vi "Get%20Printers%20Available%20and%20Setting%20a%20Default%20One%202012%20NIVerified.vi"() -> ()   [LabVIEW 2015]
uses:
  System.Drawing
  winspool.drv
panel:
  out "error out":errorcluster
  out "Printers":T1(array[cluster])
  in  "Index":i32
  # "Overview:This example shows a quick way to provide the user a list of print available and set a default one.\nRequirements:\n•\tLabVIEW 2012 (or compatible)\nInstructions:\n•\tSelect the printer number as the default one.\n•\tRun the program"
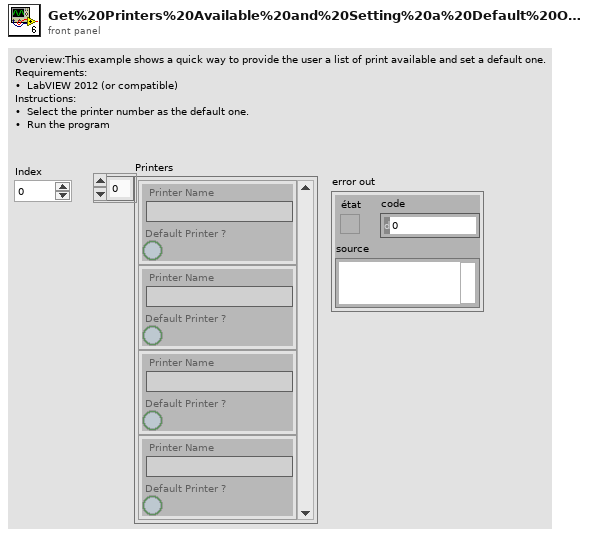
[diagram p1: front panel]
types:
  T1 = cluster{"Printer Name":string, "Default Printer ?":bool}[]
  T2 = cluster{"get_Item":string, "IsDefaultPrinter":bool}
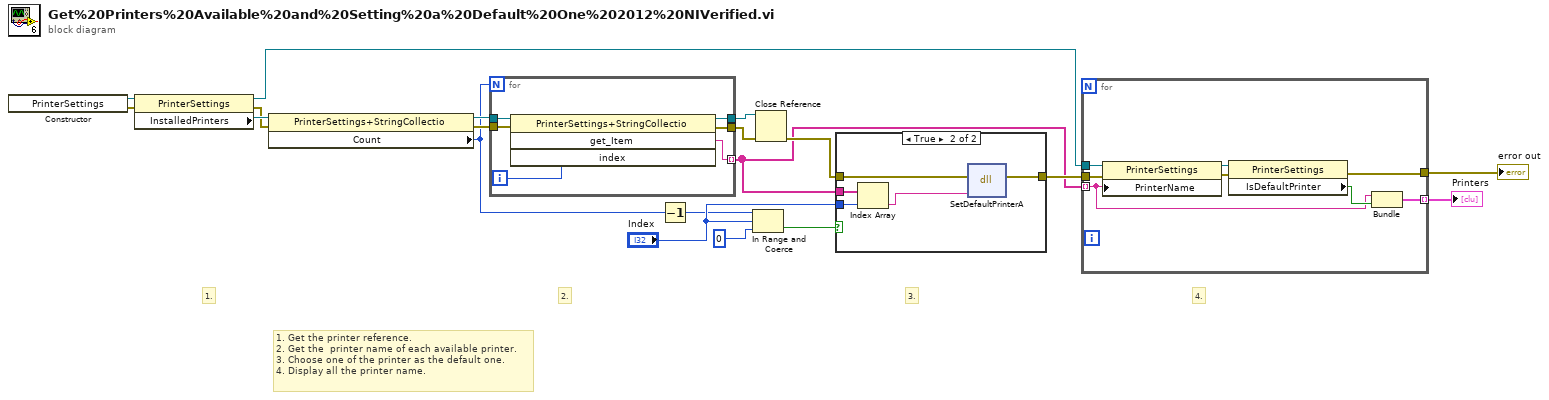
[diagram p0: block diagram]
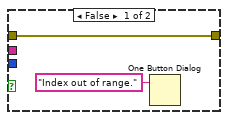
[diagram p2: hidden frame]
diagram:
  # "1. Get the printer reference.\n2. Get the  printer name of each available printer.\n3. Choose one of the printer as the default one.\n4. Display all the printer name."
  # "4."
  # "3."
  # "2."
  # "1."
  n1 = constructor class="PrinterSettings"() -> (reference out=w13:refnum<k24>, error out=w16:errorcluster)  [unwired: 3 in, 1 out]
  n2 = property class="PrinterSettings"(reference=w13, error in=w16) -> (reference out=w4:refnum<k24>, error out=w15:errorcluster, "InstalledPrinters"=w19:refnum<k24>)
  n3 = property class="PrinterSettings+StringCollectio"(reference=w19, error in=w15) -> (reference out=w17:refnum<k24>, error out=w14:errorcluster, "Count"=w7:i32)
  n4 = for {
    N: w7 -> [_]
    tunnel: w17 -> [w25]
    tunnel: [w20] -> w3 mode=indexing
    tunnel: [w23] -> w18
    tunnel: [w22] -> w12
    tunnel: w14 -> [w21]
    i -> [w24]
    n5 = invoke class="PrinterSettings+StringCollectio" method="get_Item"(reference=w25, error in=w21, "index"=w24) -> (reference out=w23:refnum<k24>, error out=w22:errorcluster, "get_Item"=w20:string)  [unwired: 1 in, 1 out]
  }
  n6 = Decrement(x=w7) -> (x-1=w8:i32)
  n7 = In Range and Coerce(upper limit=w8, x="Index", lower limit=0 ("limite inférieure")) -> (In Range?=w11:bool)  [unwired: 1 out]
  n8 = Close Reference(reference=w18, error in (no error)=w12) -> (error out=w5:errorcluster)
  n9 = case shown="True" w11 {
    tunnel: w3 -> [_ w32]
    tunnel: "Index" -> [_ w31]
    tunnel: [w26 w29] -> w6
    tunnel: w5 -> [w26 w28]
    frame False {
      n10 = One Button Dialog(message="Index out of range.") -> ()  [unwired: 1 in, 1 out]
    }
    frame True {
      n11 = Index Array(array=w32, index=w31) -> (element=w30:string)
      n12 = dll-call lib="winspool.drv" fn="SetDefaultPrinterA"(error in=w28, "pszPrinter"=w30) -> (error out=w29:errorcluster)  [unwired: 4 in, 1 out]
    }
  }
  n13 = for {
    tunnel: w6 -> [w35]
    tunnel: [w37] -> w2 mode=indexing
    tunnel: w4 -> [w36]
    tunnel: w3 -> [w34] mode=indexing
    tunnel: [w33] -> w1
    n14 = property class="PrinterSettings"(reference=w36, error in=w35, "PrinterName"=w34) -> (reference out=w40:refnum<k24>, error out=w39:errorcluster)
    n15 = property class="PrinterSettings"(reference=w40, error in=w39) -> (error out=w33:errorcluster, "IsDefaultPrinter"=w38:bool)  [unwired: 1 out]
    n16 = Bundle("get_Item"=w34, "IsDefaultPrinter"=w38) -> (w37:T2)  [unwired: 1 in]
  }
  "Printers" <- w2
  "error out" <- w1
